vi "FTW-Endpoint-Multipart-Tell.vi"(0 "FTW Endpoint":refnum<class "FTW-Endpoint.lvclass">, 5 "Message":T1, 7 "Timeout":i32 format="%dmsec", 11 "error in":errorcluster) -> (4 "FTW Endpoint out":refnum<class "FTW-Endpoint.lvclass">, 6 "Timed out?":bool, 15 "error out":errorcluster)   [LabVIEW 2013, in "FTW-Endpoint.lvclass"]
uses:
  FTW-Endpoint.lvclass
  Payload/FTW-MessagePayload.ctl
  FTW-Endpoint.lvclass/FTW-Endpoint.ctl
panel:
  # "Inputs"
  # "Outputs"
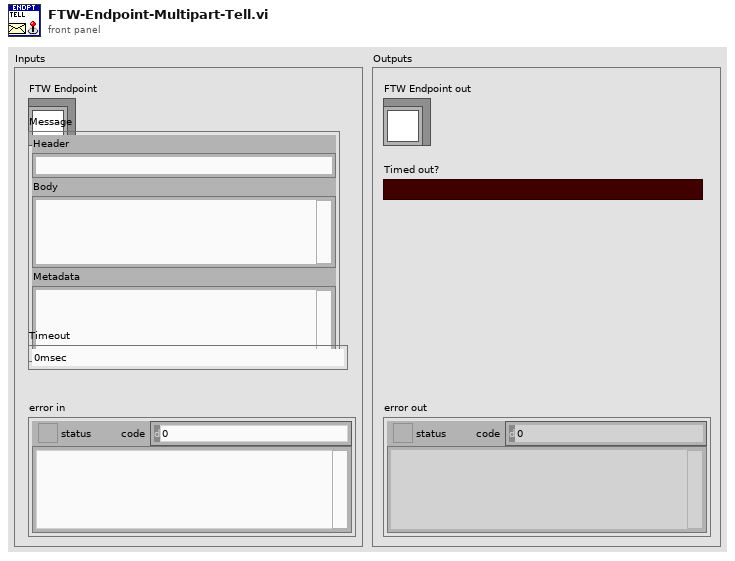
[diagram p1: front panel]
types:
  T1 = typedef "FTW-MessagePayload.ctl" = cluster{"Header":string, "Body":string, "Metadata":string}
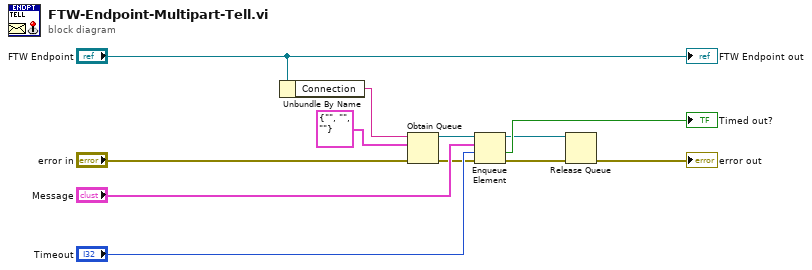
[diagram p0: block diagram]
diagram:
  n1 = Unbundle By Name("FTW Endpoint") -> ("Connection"=w4:string)
  n2 = Obtain Queue(name (unnamed)=w4, element data type=T1 {"Header"="", "Body"="", "Metadata"=""}, error in (no error)="error in") -> (queue out=w3:refnum<queue>, error out=w5:errorcluster)  [unwired: 2 in, 1 out]
  n3 = Enqueue Element(queue=w3, element="Message", timeout in ms (-1)="Timeout", error in (no error)=w5) -> (queue out=w1:refnum<queue>, timed out?=→"Timed out?":bool, error out=w6:errorcluster)
  n4 = Release Queue(queue=w1, error in (no error)=w6) -> (error out=→"error out":errorcluster)  [unwired: 1 in, 2 out]
  "FTW Endpoint out" <- "FTW Endpoint"
